vi "log from error queue.vi"() -> ()   [LabVIEW 2020]
uses:
  Error log.ctl
  Global Variables/General Globals.vi
panel:
  out "x-y":dbl
  out "Numeric":i32
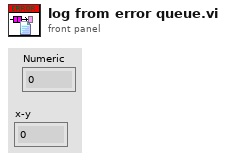
[diagram p1: front panel]
types:
  T1 = enum16{"Create/Open File", "Write File", "Close file"}
  T2 = typedef "Error log.ctl" = cluster{timestamp, string[], "error in (no error)":errorcluster}
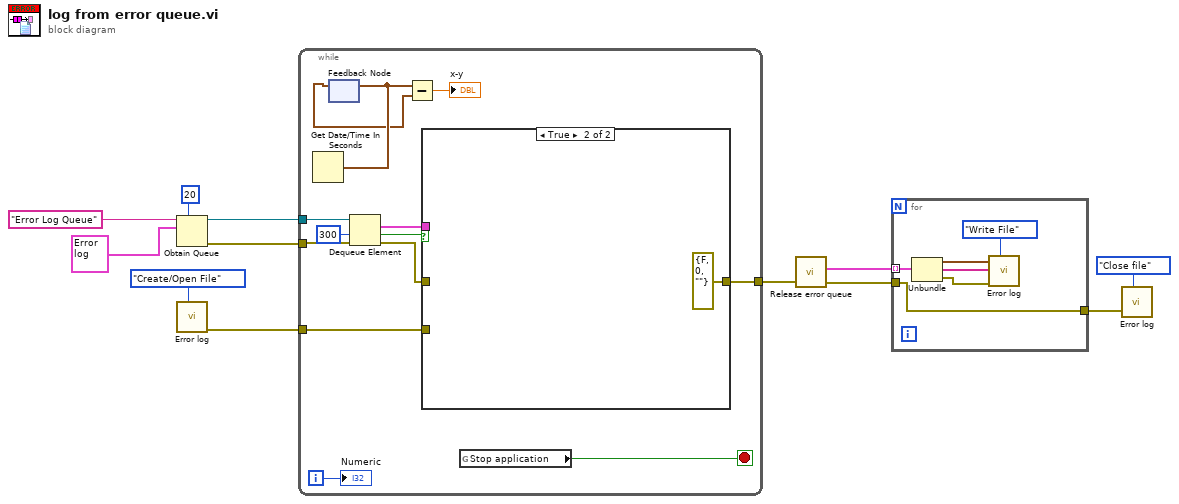
[diagram p0: block diagram]
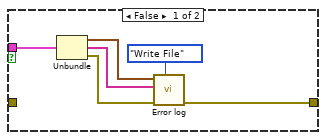
[diagram p2: hidden frame]
diagram:
  n1 = Obtain Queue(max queue size (-1, unlimited)=20, name (unnamed)="Error Log Queue", element data type=T2 {timestamp(0 s since 1904-01-01), [], "error in (no error)"={"status"=FALSE, "code"=0, "source"=""}}) -> (queue out=w8:refnum<queue>, error out=w9:errorcluster)  [unwired: 2 in, 1 out]
  n2 = call "Error log.vi"("File Ops"=T1."Create/Open File") -> ("error out 2"=w6:errorcluster)  [unwired: 10 in]
  n3 = while {
    tunnel: w9 -> [w25]
    tunnel: w8 -> [w24]
    tunnel: w6 -> [w19]
    tunnel: [w17] -> w5
    i -> [w16]
    stop <- w21 stop-if-true
    n4 = Get Date/Time In Seconds() -> (seconds since 1Jan1904=w15:timestamp)
    n5 = feedback-in #1(w15) -> ()
    n6 = feedback #1() -> (w14:timestamp)  [unwired: 1 in]
    n7 = Dequeue Element(queue=w24, timeout in ms (-1)=300, error in (no error)=w25) -> (element=w20:T2, timed out?=w22:bool, error out=w18:errorcluster)  [unwired: 1 out]
    n8 = Subtract(x=w15, y=w14) -> (x-y=→"x-y":dbl)
    n9 = case shown="True" w22 {
      tunnel: w20 -> [w30 _]
      tunnel: w19 -> [_ _]
      tunnel: [w26 errorcluster {"status"=FALSE, "code"=0, "source"=""} ("error out 2")] -> w17
      tunnel: w18 -> [_ _]
      frame False {
        n10 = Unbundle(w30) -> (w29:timestamp, w28:string[], "error in (no error)"=w27:errorcluster)
        n11 = call "Error log.vi"("File Ops"=T1."Write File", "error in (no error)"=w27, "Call Chain"=w28, "time stamp"=w29) -> ("error out 2"=w26:errorcluster)  [unwired: 7 in]
      }
      frame True {
      }
    }
    n12 = global read "General Globals.vi" "Stop application"() -> (w21:bool)
    "Numeric" <- w16
  }
  n13 = call "Release error queue.vi"("error in (no error)"=w5) -> ("error out"=w4:errorcluster, "remaining elements"=w3:T2[])  [unwired: 9 in]
  n14 = for {
    tunnel: w4 -> [w33]
    tunnel: w3 -> [w37] mode=indexing
    tunnel: [w33] -> w1
    n15 = Unbundle(w37) -> (w36:timestamp, w35:string[], "error in (no error)"=w34:errorcluster)
    n16 = call "Error log.vi"("File Ops"=T1."Write File", "error in (no error)"=w34, "Call Chain"=w35, "time stamp"=w36) -> ()  [unwired: 7 in, 1 out]
  }
  n17 = call "Error log.vi"("File Ops"=T1."Close file", "error in (no error)"=w1) -> ()  [unwired: 9 in, 1 out]
